vi "Get NI-SWITCH Description.vi"(8 "error in":errorcluster, 11 "ni-switch custom device in":T1 format="%.0x") -> (0 "error out":errorcluster, 2 "description":string, 3 "ni-switch custom device out":T1 format="%.0x")   [LabVIEW 2019, in "NI-SWITCH Scripting.lvlib"]
doc: "Returns the description for the NI-SWITCH custom device."
uses:
  NI-SWITCH Scripting.lvlib
  <vilib>/NI VeriStand/Custom Device API/Custom Device Item Ref.ctl
  <vilib>/NI VeriStand/Custom Device API/Custom Device API.lvlib
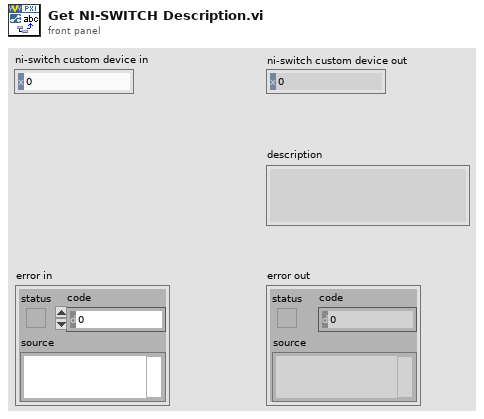
[diagram p1: front panel]
types:
  T1 = typedef "Custom Device API.lvlib/Custom Device Item Ref.ctl" = u64
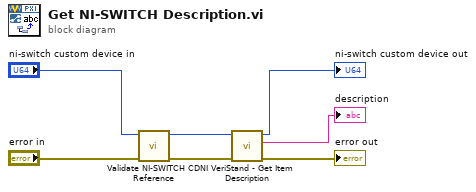
[diagram p0: block diagram]
diagram:
  n1 = call "Validate NI-SWITCH CD Reference.vi"("error in"="error in", "ni-switch custom device in"="ni-switch custom device in") -> ("error out"=w3:errorcluster, "ni-switch custom device out"=w1:T1)  [unwired: 8 in]
  n2 = call <vilib>:"NI VeriStand - Get Item Description.vi"("error in (no error)"=w3, "Item Ref in"=w1) -> ("error out"=→"error out":errorcluster, "Description"=→"description":string, "Item Ref out"=→"ni-switch custom device out":T1)  [unwired: 6 in, 1 out]
